vi "WebcamMultiplePhotos.vi"() -> ()   [LabVIEW 2017]
uses:
  <vilib>/userdefined/High Color/IMAQdx.ctl
  <vilib>/vision/driver/IMAQdx.llb/IMAQdx Camera Control Mode.ctl
  <vilib>/vision/driver/NI_Vision_Acquisition_Software.lvlib
panel:
  in  "stop 2":bool
  in  "Snap":bool
  out "x":dbl
  out "created path":path
  in  "error in":errorcluster
  in  "Image Type":T1 items=["Grayscale (U8)", "Grayscale (I16)", "Grayscale (SGL)", "Complex (CSG)", "RGB (U32)", "HSL (U32)", "RGB (U64)", "Grayscale (U16)"]
  out "error out":errorcluster
  in  "Session In":T2
  in  "stop":bool
  out "Image":T3(plugin-control)
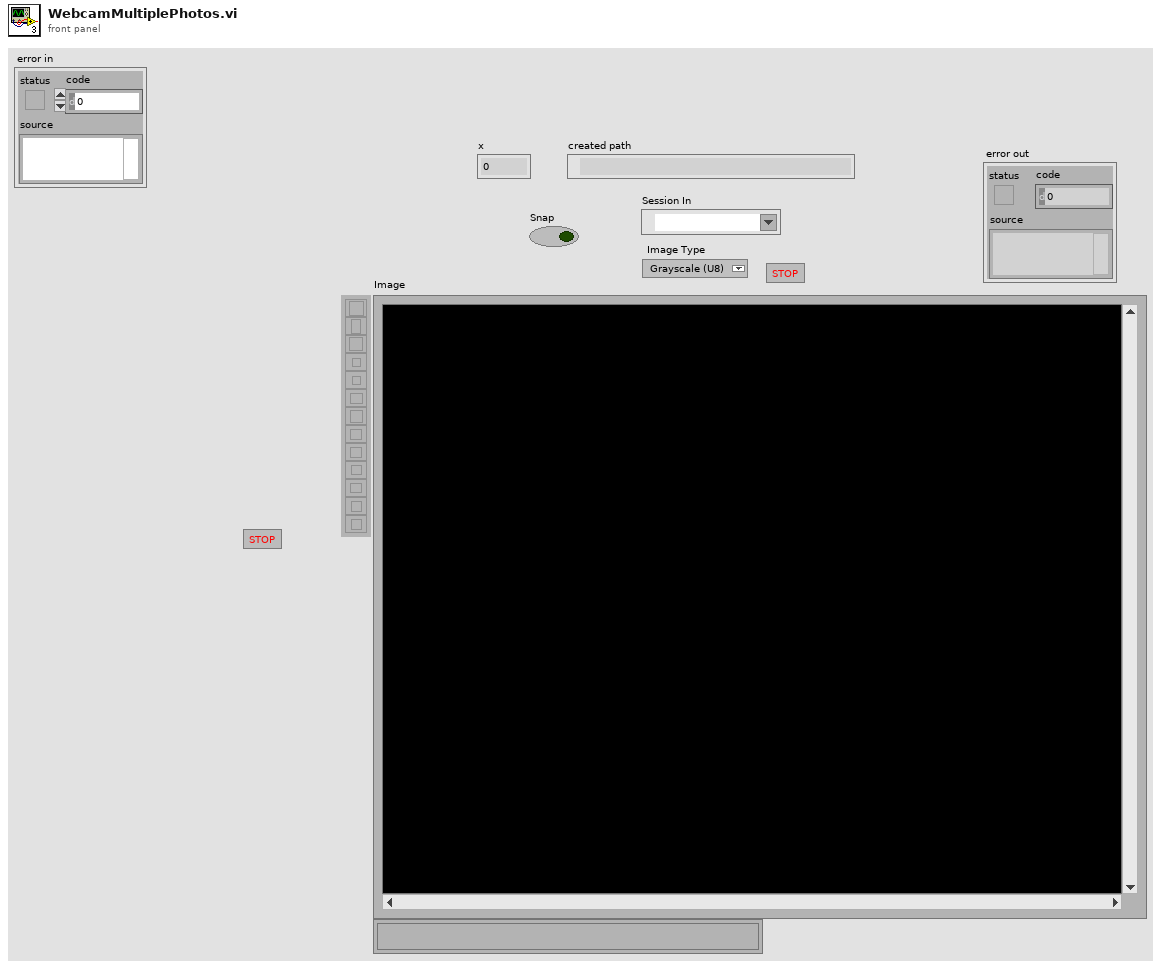
[diagram p1: front panel]
types:
  T1 = typedef "Image Type" = u32
  T2 = typedef "IMAQdx.ctl" = refnum<k21>
  T3 = typedef "IMAQ Image.ctl" = refnum<image>
  T4 = typedef "NI_Vision_Acquisition_Software.lvlib/IMAQdx Camera Control Mode.ctl" = enum32{"Controller", "Listener"}
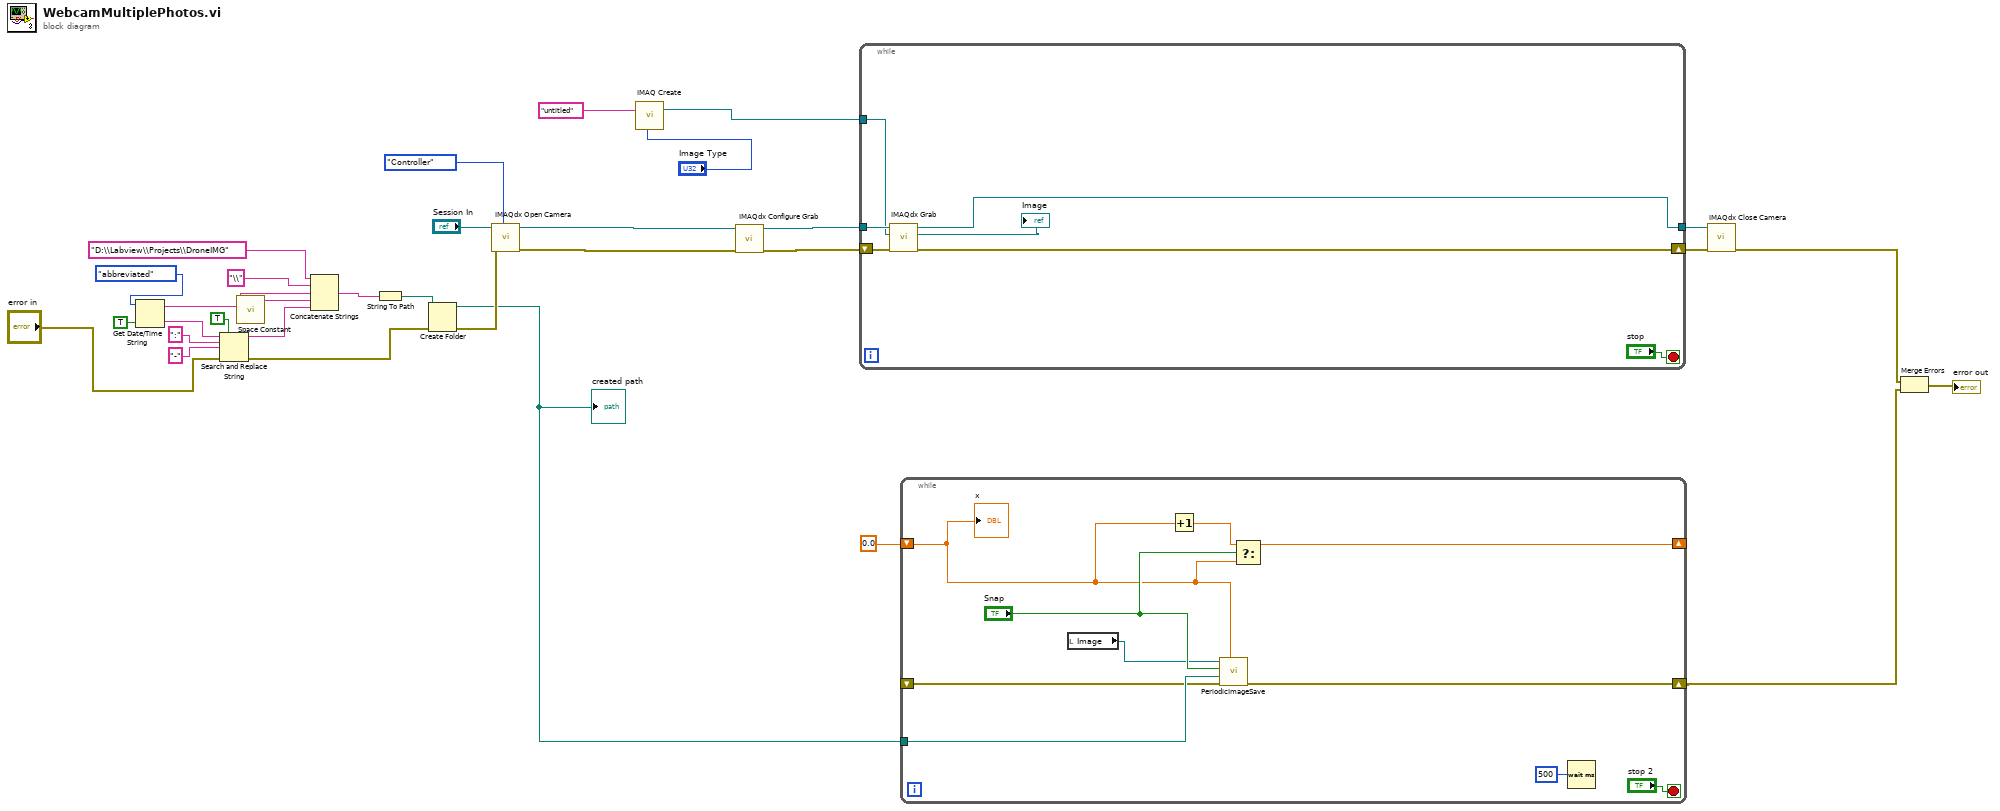
[diagram p0: block diagram]
diagram:
  n1 = Get Date/Time String(date format (0)=enum16{"short", "long", "abbreviated"}."abbreviated", want seconds? (F)=TRUE) -> (date string=w26:string, time string=w23:string)  [unwired: 1 in]
  n2 = Search and Replace String(replace all?=TRUE ("replace all? (F)"), input string=w23, search string=":" ("replace string (\"\")"), replace string="-" ("replace string (\"\")"), error in="error in") -> (result string=w24:string, error out=w12:errorcluster)  [unwired: 3 in, 2 out]
  n3 = call <vilib>:"Space Constant.vi"() -> ("String"=w25:string)
  n4 = Concatenate Strings("D:\\Labview\\Projects\\DroneIMG" ("string"), "\\" ("string"), w26, w25, w24) -> (w15:string)
  n5 = String To Path(string=w15) -> (path=w14:path)
  n6 = Create Folder(path (use dialog)=w14, error in=w12) -> (created path=w10:path, error out=w11:errorcluster)  [unwired: 1 in, 1 out]
  "created path" <- w10
  n7 = call <vilib>:"IMAQdx Open Camera.vi"("Camera Control Mode"=IMAQdx_Camera_Control_Mode."Controller", "error in"=w11, "Session In"="Session In") -> ("error out"=w2:errorcluster, "Session Out"=w31:T2)  [unwired: 7 in]
  n8 = call "IMAQ Create"("Image Name"="untitled", "Image Type"="Image Type") -> ("New Image"=w5:T3)  [unwired: 3 in, 1 out]
  n9 = call <vilib>:"IMAQdx Configure Grab.vi"("error in"=w2, "Session In"=w31) -> ("error out"=w1:errorcluster, "Session Out"=w30:T2)  [unwired: 8 in]
  n10 = while {
    tunnel: w30 -> [w38]
    tunnel: [w36] -> w27
    shift-right: [w33] -> w7
    shift-left: w1 -> [w37]
    tunnel: w5 -> [w35]
    stop <- "stop" stop-if-true
    n11 = call <vilib>:"IMAQdx Grab.vi"("error in"=w37, "Image In"=w35, "Session In"=w38) -> ("error out"=w33:errorcluster, "Image Out"=→"Image":T3, "Session Out"=w36:T2)  [unwired: 5 in, 1 out]
  }
  n12 = while {
    shift-right: [w43] -> _
    shift-left: 0.0 -> [w44]
    tunnel: w10 -> [w47]
    shift-right: [w40] -> w6
    shift-left: _ -> [w41]
    stop <- "stop 2" stop-if-true
    n13 = local read "Image"() -> (w42:T3)
    n14 = Increment(x=w44) -> (x+1=w45:dbl)
    n15 = call "PeriodicImageSave.vi"("x"=w44, "error in (no error)"=w41, "in path"=w47, "Snap"="Snap", "Image In"=w42) -> ("error out"=w40:errorcluster)  [unwired: 5 in]
    n16 = Select(t=w45, s="Snap", f=w44) -> (s? t:f=w43:dbl)
    n17 = Wait (ms)(milliseconds to wait=u32 500) -> ()  [unwired: 1 out]
    "x" <- w44
  }
  n18 = call <vilib>:"IMAQdx Close Camera.vi"("error in"=w7, "Session In"=w27) -> ("error out"=w4:errorcluster)  [unwired: 9 in]
  n19 = Merge Errors(w4, w6) -> (→"error out":errorcluster)
